vi "Set Report Margins.vi"(0 "report in":refnum<class "NI_Standard Report.lvclass">, 5 "margins (1.00)":T1={"top"=1.0, "left"=1.0, "right"=1.0, "bottom"=1.0} {"right" format="%.2f"; "bottom" format="%.2f"; "top" format="%.2f"; "left" format="%.2f"}, 9 "measurement system (default)":u16(ring) items=["Default", "US", "Metric"], 11 "error in (no error)":errorcluster) -> (4 "report out":refnum<class "NI_Standard Report.lvclass">, 10 "page width (Word)":sgl format="%.2f", 15 "error out":errorcluster)   [LabVIEW 2015, in "NI_Standard Report.lvclass"]
doc: "Sets the margins of the specified report."
uses:
  <vilib>/Utility/NIReport.llb/Standard Report/NI_Standard Report.lvclass
  <vilib>/Utility/NIReport.llb/Standard Report/NI_Standard Report.lvclass/NI_Standard Report.ctl
  <vilib>/Utility/NIReport.llb/NI_ReportGenerationCore.lvlib
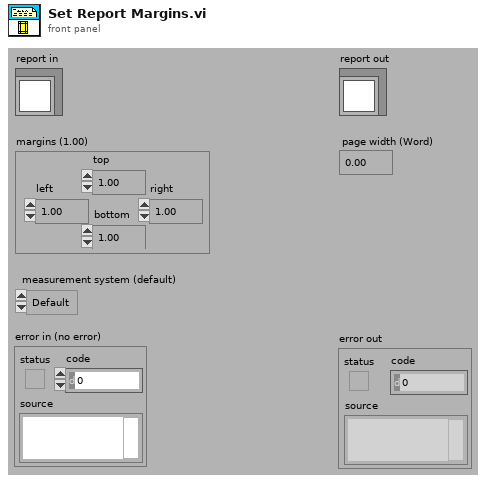
[diagram p1: front panel]
types:
  T1 = cluster{"top":dbl, "left":dbl, "right":dbl, "bottom":dbl}
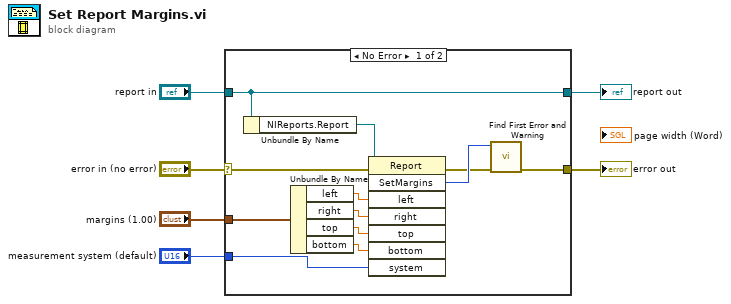
[diagram p0: block diagram]
diagram:
  n1 = case shown="No Error" "error in (no error)" {
    selector: "error in (no error)" -> [w8 w20]
    tunnel: [w7 w20] -> w5
    tunnel: [w11 w19] -> w3
    tunnel: "report in" -> [w11 w19]
    tunnel: "margins (1.00)" -> [w10 _]
    tunnel: "measurement system (default)" -> [w9 _]
    frame No Error {
      n2 = Unbundle By Name(w11) -> ("NIReports.Report"=w14:refnum<k7>)
      n3 = Unbundle By Name(w10) -> ("left"=w15:dbl, "right"=w16:dbl, "top"=w17:dbl, "bottom"=w18:dbl)
      n4 = invoke class="Report" method="SetMargins"(reference=w14, error in=w8, "left"=w15, "right"=w16, "top"=w17, "bottom"=w18, "system"=w9) -> (error out=w12:errorcluster, "SetMargins"=w13:i32)  [unwired: 1 in, 6 out]
      n5 = call <vilib>:"Find First Error and Warning.vi"("error in (no error)"=w12, "error code"=w13) -> ("error out"=w7:errorcluster)  [unwired: 1 in, 4 out]
    }
    frame Error {
    }
  }
  "error out" <- w5
  "report out" <- w3
